vi "Config Globals.vi"() -> ()   [LabVIEW 2015, in "Config Module.lvlib"]
uses:
  Config Module.lvlib
  Controls/Config Cluster.ctl
  Controls/Vision Config Cluster.ctl
  Transport/Controls/Transport XML Cluster.ctl
  MTI/Public Controls/Operation Mode enum.ctl
  Profile Module/Controls/MTI Parameter Settings.ctl
  Profile Module/Controls/Profile Measure By Enum.ctl
  MTI/Public Controls/MTI Measure enum.ctl
  Height Measurement Module/Public Controls/HM-Settings Cluster.ctl
  Diameter Module/Controls/PreConditioning Settings Cluster.ctl
  Diameter Module/Controls/Diameter Processing Settings Cluster.ctl
panel:
  out "Config":T1={"Vision"={"Exposure Time (us)"=1, "Full Frame Rate"=1.0, "Allowed Part Time (s)"=0.024, "Save Bad Images"=FALSE, "max tries"=0}, "Transport XML Cluster"={"Galil IP address"="192.168.70.13", "settle time (ms)"=0}, "MTI_1"={"IP_Address"="192.168.70.13", "Sensor"=1, "Mode"=enum."Real", "VideoGain"=0.0, "LaserIntensity"=0.0, "Scans"=1, "reverse scan"=TRUE}, "MTI_2"={"IP_Address"="192.168.70.11", "Sensor"=1, "Mode"=enum."Real", "VideoGain"=0.0, "LaserIntensity"=127.0, "Scans"=1, "reverse scan"=FALSE}, "Parts Timeout (min)"=60.0, "Profile Measure Settings"={"lower limit outliers range (in)"=0.2, "upper limit outliers range (in)"=0.2, "Measure By"=enum."Minimum", "Measure.Minimum Drop Samples"=15, "Measure"=enum."Height", "Min Intensity Threshold"=50, "Z Height Threshold Fraction"=0.35, "Min Z Threshold (mm)"=1.5, "Laser 1 offset (inch)"=0.0, "Laser 1 gain"=0.0, "Laser 2 offset (inch)"=0.0, "Laser 2 gain"=0.0, "Zero Biggest N Points"=0}, "Divert Period (min)"=60.0, "Diameter Processing Settings"={"PreConditioning Settings"={"small particle max intensity"=190, "small particle max area (pixels)"=5000}}, "MTI DLL path"=path "", "Force Parts to Pass"=FALSE, "Save Bad Laser Profiles"=FALSE} {"Profile Measure Settings"."Min Z Threshold (mm)" format="%#_13g"; "Profile Measure Settings"."Z Height Threshold Fraction" format="%#_13g"; "Profile Measure Settings"."upper limit outliers range (in)" format="%#_13g"; "Profile Measure Settings"."lower limit outliers range (in)" format="%#_13g"; "MTI_2"."Scans" min=1 max=90; "MTI_2"."LaserIntensity" min=0.0 max=127.0; "MTI_2"."VideoGain" min=0.0 max=1023.0; "MTI_2"."Sensor" min=1 max=5; "MTI_1"."Scans" min=1 max=90; "MTI_1"."LaserIntensity" min=0.0 max=127.0; "MTI_1"."VideoGain" min=0.0 max=1023.0; "MTI_1"."Sensor" min=1 max=5}
  # "Nate disconnected the Board ID and Axis / Vector Space from the typedef\nbecause NI-Motion is not availabe in 64-bit"
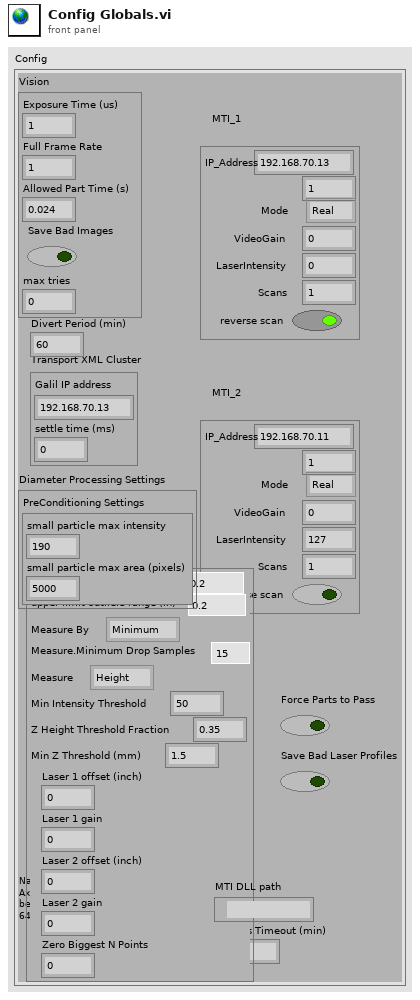
[diagram p1: front panel]
types:
  T1 = typedef "Config Module.lvlib/Config Cluster.ctl" = cluster{"Vision":T2, "Transport XML Cluster":T3, "MTI_1":T4, "MTI_2":T4, "Parts Timeout (min)":dbl, "Profile Measure Settings":T6, "Divert Period (min)":dbl, "Diameter Processing Settings":T9, "MTI DLL path":path, "Force Parts to Pass":bool, "Save Bad Laser Profiles":bool}
  T2 = typedef "Config Module.lvlib/Vision Config Cluster.ctl" = cluster{"Exposure Time (us)":i32, "Full Frame Rate":dbl, "Allowed Part Time (s)":dbl, "Save Bad Images":bool, "max tries":i32}
  T3 = typedef "Transport.lvclass/Transport XML Cluster.ctl" = cluster{"Galil IP address":string, "settle time (ms)":i32}
  T4 = typedef "MTI Parameter Settings.ctl" = cluster{"IP_Address":string, "Sensor":i32, "Mode":T5, "VideoGain":dbl, "LaserIntensity":dbl, "Scans":i32, "reverse scan":bool}
  T5 = typedef "MTI Module.lvlib/MTI.lvclass/Operation Mode enum.ctl" = enum16{"Real", "Sim"}
  T6 = typedef "HM-Settings Cluster.ctl" = cluster{"lower limit outliers range (in)":dbl, "upper limit outliers range (in)":dbl, "Measure By":T7, "Measure.Minimum Drop Samples":u16, "Measure":T8, "Min Intensity Threshold":i32, "Z Height Threshold Fraction":dbl, "Min Z Threshold (mm)":dbl, "Laser 1 offset (inch)":dbl, "Laser 1 gain":dbl, "Laser 2 offset (inch)":dbl, "Laser 2 gain":dbl, "Zero Biggest N Points":i32}
  T7 = typedef "Profile Measure By Enum.ctl" = enum16{"Mode", "Minimum"}
  T8 = typedef "MTI Module.lvlib/MTI.lvclass/MTI Measure enum.ctl" = enum16{"Height", "Depth"}
  T9 = typedef "Diameter Module Library.lvlib/Diameter Processing Settings Cluster.ctl" = cluster{"PreConditioning Settings":T10}
  T10 = typedef "Diameter Module Library.lvlib/PreConditioning Settings Cluster.ctl" = cluster{"small particle max intensity":i32, "small particle max area (pixels)":i32}
diagram:
